vi "RESPALDO.vi"() -> ()   [LabVIEW 2017]
uses:
  <vilib>/myRIO/Instrument Drivers/Onboard IO/PWM/typedefs/PWM Reference.ctl
  <vilib>/myRIO/Common/Instrument Driver Framework/Utilities/typedefs/myRIO Generic Hardware Reference.ctl
  <vilib>/myRIO/Common/Instrument Driver Framework/Utilities/typedefs/Hardware Version Enum.ctl
  <vilib>/myRIO/Common/Instrument Driver Framework/Utilities/typedefs/myRIO v1.0 Reference.ctl
  <vilib>/myRIO/Common/Instrument Driver Framework/Utilities/typedefs/Generic FPGA Reference.ctl
  <vilib>/myRIO/Common/Instrument Driver Framework/myRIO v1.0/PWM/typedefs/PWM Channels Enum.ctl
  <vilib>/myRIO/Instrument Drivers/Onboard IO/PWM/typedefs/PWM Configuration.ctl
  <vilib>/userdefined/High Color/nirio_resource_hc.ctl
  <vilib>/myRIO/Instrument Drivers/Onboard IO/DIO/typedefs/DIO Reference.ctl
  <vilib>/myRIO/Common/Instrument Driver Framework/myRIO v1.0/DIO/typedefs/DIO Channels List.ctl
  <vilib>/myRIO/Common/Instrument Driver Framework/myRIO v1.0/DIO/typedefs/DIO Channels Enum.ctl
  <vilib>/myRIO/Common/Instrument Driver Framework/Utilities/vis/Is FPGA Ref Available.vi
  <vilib>/myRIO/Common/Instrument Driver Framework/myRIO v1.0/DIO/vis/myRIO v1.1 Open DIO.vi
  <vilib>/myRIO/Instrument Drivers/Onboard IO/DIO/vis/Write.vi
  <vilib>/myRIO/Common/Instrument Driver Framework/myRIO v1.0/PWM/vis/myRIO v1.1 Open PWM.vi
  <vilib>/myRIO/Common/Instrument Driver Framework/myRIO v1.0/UART/vis/myRIO v1.0 Close UART.vi
  <vilib>/myRIO/Common/Instrument Driver Framework/Utilities/vis/Validate Channels.vi
  <vilib>/myRIO/Common/Instrument Driver Framework/myRIO v1.0/DIO/vis/myRIO v1.0 Reserve DIO.vi
  <vilib>/myRIO/Common/Instrument Driver Framework/myRIO v1.0/PWM/vis/myRIO v1.0 Reserve PWM.vi
  <vilib>/myRIO/Common/Instrument Driver Framework/myRIO v1.0/Resource Manager/vis/myRIO v1.0 Reserve Channel List.vi
  <vilib>/myRIO/Common/Instrument Driver Framework/myRIO v1.0/DIO/vis/myRIO v1.0 Build MUX Configuration DIO.vi
  <vilib>/myRIO/Common/Instrument Driver Framework/myRIO v1.0/PWM/vis/myRIO v1.0 Build MUX Configuration PWM.vi
  <vilib>/myRIO/Common/Instrument Driver Framework/myRIO v1.0/Resource Manager/vis/myRIO v1.0 Reserve Channel.vi
  <vilib>/myRIO/Common/Instrument Driver Framework/myRIO v1.0/Resource Manager/vis/myRIO v1.0 Unreserve Channel.vi
  <vilib>/myRIO/Common/Instrument Driver Framework/myRIO v1.0/Resource Manager/vis/myRIO v1.0 Create Configuration List.vi
  <vilib>/myRIO/Common/Instrument Driver Framework/myRIO v1.0/Resource Manager/vis/myRIO v1.0 Build Mutex Name.vi
  <vilib>/Utility/VariantDataType/GetNumericInfo.vi
  <vilib>/Utility/error.llb/Error Cluster From Error Code.vi
  <vilib>/myRIO/Common/Instrument Driver Framework/myRIO v1.0/myRIO v1.1 Open.vi
  <vilib>/myRIO/Common/Instrument Driver Framework/Utilities/vis/IO Manager.vi
  <vilib>/myRIO/Common/Instrument Driver Framework/Utilities/vis/Configuration Manager.vi
  <vilib>/myRIO/Common/Instrument Driver Framework/myRIO v1.0/Resource Manager/vis/myRIO v1.0 Configure IO.vi
  <vilib>/myRIO/Common/Instrument Driver Framework/myRIO v1.0/myRIO v1.0 Close.vi
  <vilib>/myRIO/Common/Instrument Driver Framework/myRIO v1.0/PWM/vis/myRIO v1.0 Write PWM.vi
  <vilib>/myRIO/Common/Instrument Driver Framework/myRIO v1.0/DIO/vis/myRIO v1.0 Write DIO.vi
  <vilib>/myRIO/Common/Instrument Driver Framework/Utilities/vis/FPGA Ref Manager.vi
  <vilib>/myRIO/Common/Instrument Driver Framework/myRIO v1.0/myRIO v1.0 Reset FPGA.vi
  <vilib>/myRIO/Common/Instrument Driver Framework/myRIO v1.0/IRQ/vis/myRIO v1.0 IRQ Info FGV.vi
  <vilib>/myRIO/Common/Instrument Driver Framework/myRIO v1.0/IRQ/vis/myRIO v1.0 Timer IRQ Info FGV.vi
  <vilib>/myRIO/Common/Instrument Driver Framework/myRIO v1.0/IRQ/vis/myRIO v1.0 ISR Agent.vi
  <vilib>/myRIO/Express VI/Onboard IO/PWM/PWM Express VI.xnode
  <vilib>/myRIO/Instrument Drivers/Onboard IO/PWM/vis/myRIO PWM Open.xnode
  <vilib>/myRIO/Express VI/Onboard IO/DO/DO Express VI.xnode
  <vilib>/myRIO/Instrument Drivers/Onboard IO/DIO/vis/myRIO DIO Open.xnode
  <vilib>/myRIO/Instrument Drivers/Utilities/Utilities.lvlib
  <vilib>/myRIO/Instrument Drivers/Onboard IO/PWM/PWM.lvlib
  <vilib>/myRIO/Instrument Drivers/Onboard IO/DIO/DIO.lvlib
panel:
  in  "delta":dbl
  in  "Numeric 7":dbl
  in  "Numeric 6":dbl
  out "Numeric 5":dbl
  out "Numeric 4":dbl
  out "Numeric 3":dbl
  in  "MODO JOG":bool
  out "Numeric 2":dbl
  out "Slide 2":dbl(slide) scale=-200.0..100.0
  out "Slide":dbl(slide) scale=-200.0..100.0
  out "Numeric":dbl
  in  "control":T1(tab)
  in  "PARADA":bool
  out "ESTADO":string
  in  "?":bool
  out "MODO":string
  in  "Boolean":bool
  in  "PWM channel":tag="B/PWM0"
  in  "PWM channel 2":tag="B/PWM0"
  out "offset [%FS] 3":dbl
  in  "null offset 3":bool
  out "duty cycle [%] 3":dbl
  out "pulse width [ms] 3":dbl=1.5
  in  "position 2":dbl(slide) scale=-200.0..200.0
  in  "PWM channel 3":tag="B/PWM0"
  out "offset [%FS] 4":dbl
  in  "null offset 4":bool
  out "duty cycle [%] 4":dbl
  out "pulse width [ms] 4":dbl=1.5
  in  "position [%FS] 4":dbl(slide) scale=-200.0..200.0
  out "offset [%FS] 5":dbl
  in  "null offset 5":bool
  out "duty cycle [%] 5":dbl
  out "pulse width [ms] 5":dbl=1.5
  in  "position [%FS] 5":dbl(slide) scale=-200.0..200.0
  out "position [%FS]":dbl
  out "position [3":dbl
  out "position1":dbl
  out "ventosa":bool
  out "POSICION1":dbl
  out "POSICION2":dbl
  out "POSICION3":dbl
  in  "velocidad":dbl(knob) scale=20.0..250.0
  in  "PARADA":bool
  out "INDICADOR 2":bool
  out "INDICADOR1":bool
  in  "PARADA":bool
  in  ".":dbl(slide) scale=0.0..10.0
  in  ".":dbl(slide) scale=0.0..10.0
  out "String":string
  out "CADENA1":dbl
  out "CADENA2":dbl
  in  "Puero de servicio remoto":u16
  in  "direccion":string
  in  "PARADA":bool
  out "Datos recibidos vía TCP":cluster{dbl, dbl}(graph)
  out "offset [%FS] 2":dbl
  in  "null offset 2":bool
  out "duty cycle [%] 2":dbl
  out "pulse width [ms] 2":dbl=1.5
  in  "freq [Hz] 2":dbl=50.0
  in  "position [%FS] 3":dbl(slide) scale=-400.0..400.0
  in  "PWM channel 6":tag="B/PWM0"
  in  "PWM channel 5":tag="B/PWM0"
  in  "position [%FS] 2":dbl(slide) scale=-400.0..400.0
  in  "freq [Hz]":dbl=50.0
  out "pulse width [ms]":dbl=1.5
  out "duty cycle [%]":dbl
  in  "null offset":bool
  out "offset [%FS]":dbl
  out "offset [%FS] 6":dbl
  in  "null offset 6":bool
  out "duty cycle [%] 6":dbl
  out "pulse width [ms] 6":dbl=1.5
  in  "freq [Hz] 3":dbl=50.0
  in  "position [%FS] 6":dbl(slide) scale=-400.0..400.0
  in  "PWM channel 7":tag="B/PWM0"
  in  "VELOCIDAD1":dbl(knob) scale=0.0..1.0
  in  "VELOCIDAD 2":dbl(knob) scale=0.0..1.0
  in  "DIRECCION1":bool
  in  "DIRECCION 2":bool
  in  "servomotores":bool
  out "V1":dbl
  out "V2":dbl
  # "BIENVENIDOS A LA\nINTERFAZ DE CONTROL ROBOT DELTA"
  # "INICIO DE PROCESO"
  # "SISTEMA DE ESTADO DE ROBOT DELTA"
  # "SERVOMOTOR1"
  # "SERVOMOTOR2"
  # "SERVOMOTOR3"
  # "VISUALIZACION DE CINTAS TRANSPORTADORAS"
  # "CINTA TRANSPORTADORA1"
  # "CINTA TRANSPORTADORA2"
  # "COMUNICACION CON EL SISTEMA DE VISION"
  # "DATOS DE COMIUNICACION"
  # "VISUALIZACION DE POSCICION"
  # "SERVOMOTOR1"
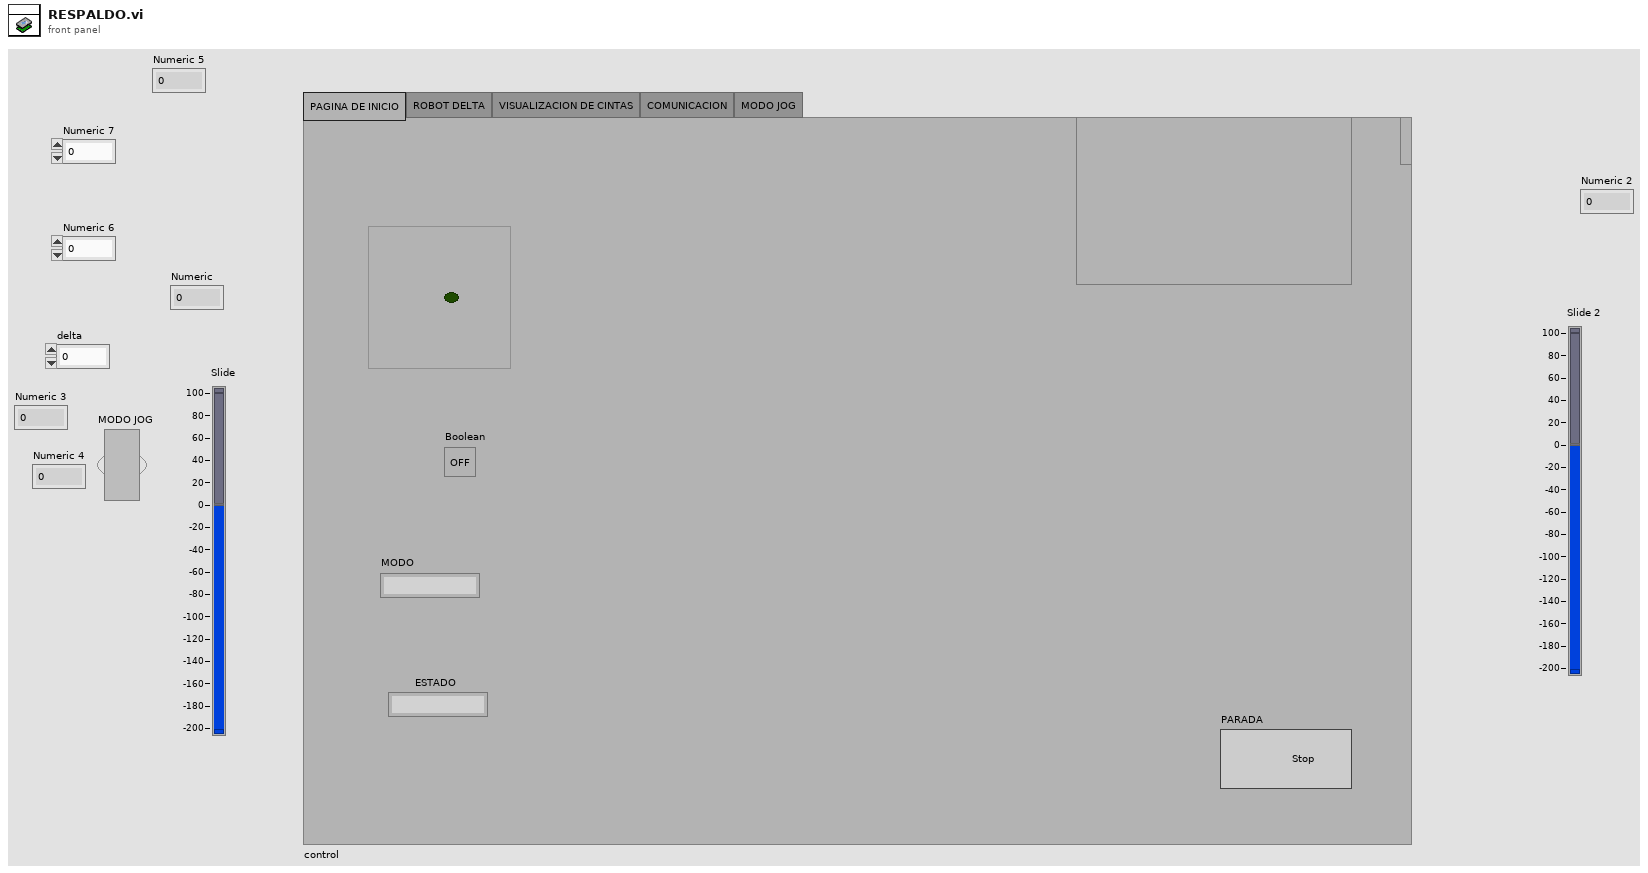
[diagram p1: front panel]
types:
  T1 = enum32{"PAGINA DE INICIO", "ROBOT DELTA", "VISUALIZACION DE CINTAS", "COMUNICACION", "MODO JOG"}
  T2 = enum16{"", "INICIO", "STOP", "DETECCION", "ESPERA", "MOVIMIENTO"}
  T3 = typedef "PWM.lvlib/PWM Reference.ctl" = cluster{"myRIO Reference":T4, "PWM Channels Enum":T8, "PWM Configuration":T9}
  T4 = typedef "myRIO Generic Hardware Reference.ctl" = cluster{"myRIO Model":T5, "myRIO Hardware Reference":T6}
  T5 = typedef "Hardware Version Enum.ctl" = enum16{"Unknown", "myRIO-1900", "myRIO-1950", "roboRIO", "NI ELVIS RIO CM"}
  T6 = typedef "myRIO v1.0 Reference.ctl" = cluster{"Generic FPGA Reference":T7, "Allow multiple opens":bool}
  T7 = typedef "Generic FPGA Reference.ctl" = refnum<k20>
  T8 = typedef "PWM Channels Enum.ctl" = enum16{"Not Connected", "C/PWM0", "C/PWM1", "A/PWM0", "A/PWM1", "A/PWM2", "B/PWM0", "B/PWM1", "B/PWM2", "PWM/PWM0", "PWM/PWM1", "PWM/PWM2", "PWM/PWM3", "PWM/PWM4", "PWM/PWM5", "PWM/PWM6", "PWM/PWM7", "PWM/PWM8", "PWM/PWM9"}
  T9 = typedef "PWM.lvlib/PWM Configuration.ctl" = cluster{"Frequency":dbl, "Duty Cycle":dbl}
  T10 = enum16{"Standard", "Buffered", "CRLF", "Immediate"}
  T11 = typedef "nirio_resource_hc.ctl" = tag
  T12 = typedef "DIO.lvlib/DIO Reference.ctl" = cluster{"myRIO Reference":T4, "DIO Channels List":T13}
  T13 = typedef "DIO Channels List.ctl" = T14[]
  T14 = typedef "DIO Channels Enum.ctl" = enum16{"Not Connected", "C/DIO0", "C/DIO1", "C/DIO2", "C/DIO3", "C/DIO4", "C/DIO5", "C/DIO6", "C/DIO7", "A/DIO0", "A/DIO1", "A/DIO2", "A/DIO3", "A/DIO4", "A/DIO5", "A/DIO6", "A/DIO7", "A/DIO8", "A/DIO9", "A/DIO10", "A/DIO11", "A/DIO12", "A/DIO13", "A/DIO14", "A/DIO15", "B/DIO0", "B/DIO1", "B/DIO2", "B/DIO3", "B/DIO4", "B/DIO5", "B/DIO6", "B/DIO7", "B/DIO8", "B/DIO9", "B/DIO10", "B/DIO11", "B/DIO12", "B/DIO13", "B/DIO14", "B/DIO15", "LED0", "LED1", "LED2", "LED3", "Button0", "DIO/DIO0", "DIO/DIO1", "DIO/DIO2", "DIO/DIO3", "DIO/DIO4", "DIO/DIO5", "DIO/DIO6", "DIO/DIO7", "DIO/DIO8", "DIO/DIO9", "SPI/CS0", "SPI/CS1", "SPI/CS2", "SPI/CS3", "LED RADIO (Green)", "LED RADIO (Red)", "LED COMM (Green)", "LED COMM (Red)", "LED MODE (Green)", "LED MODE (Red)"}
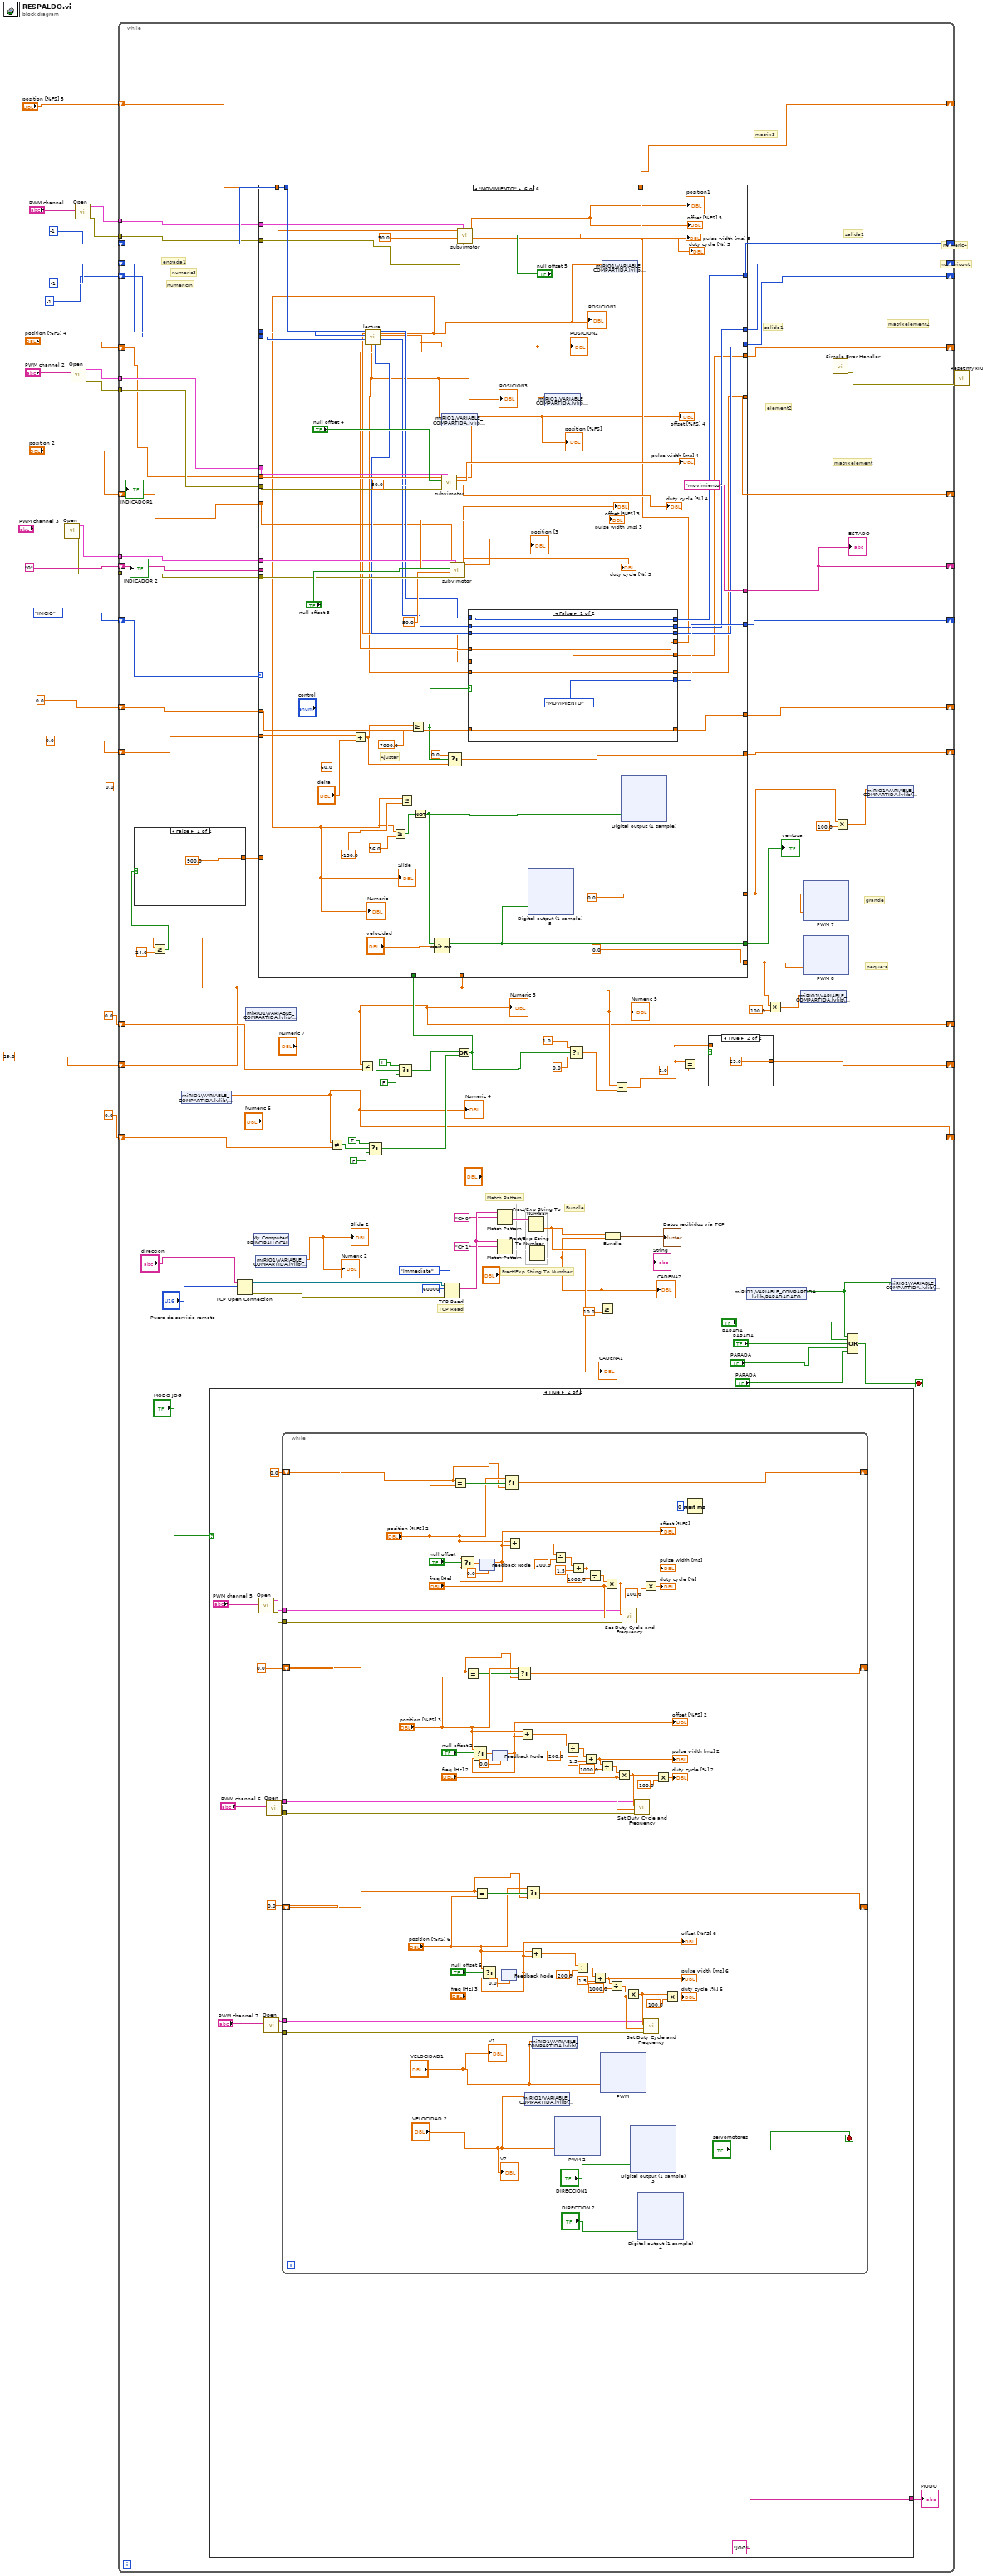
[diagram p0: block diagram]
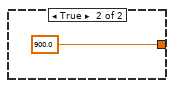
[diagram p2: hidden frame]
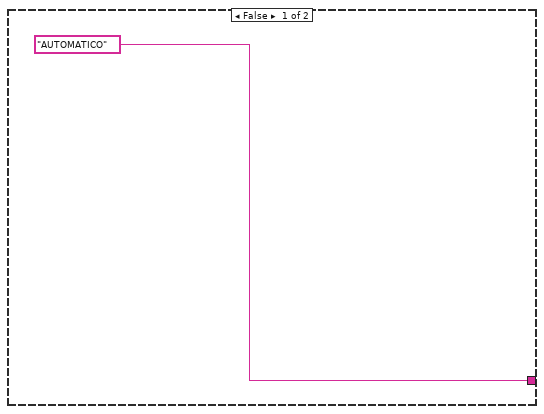
[diagram p4: hidden frame]
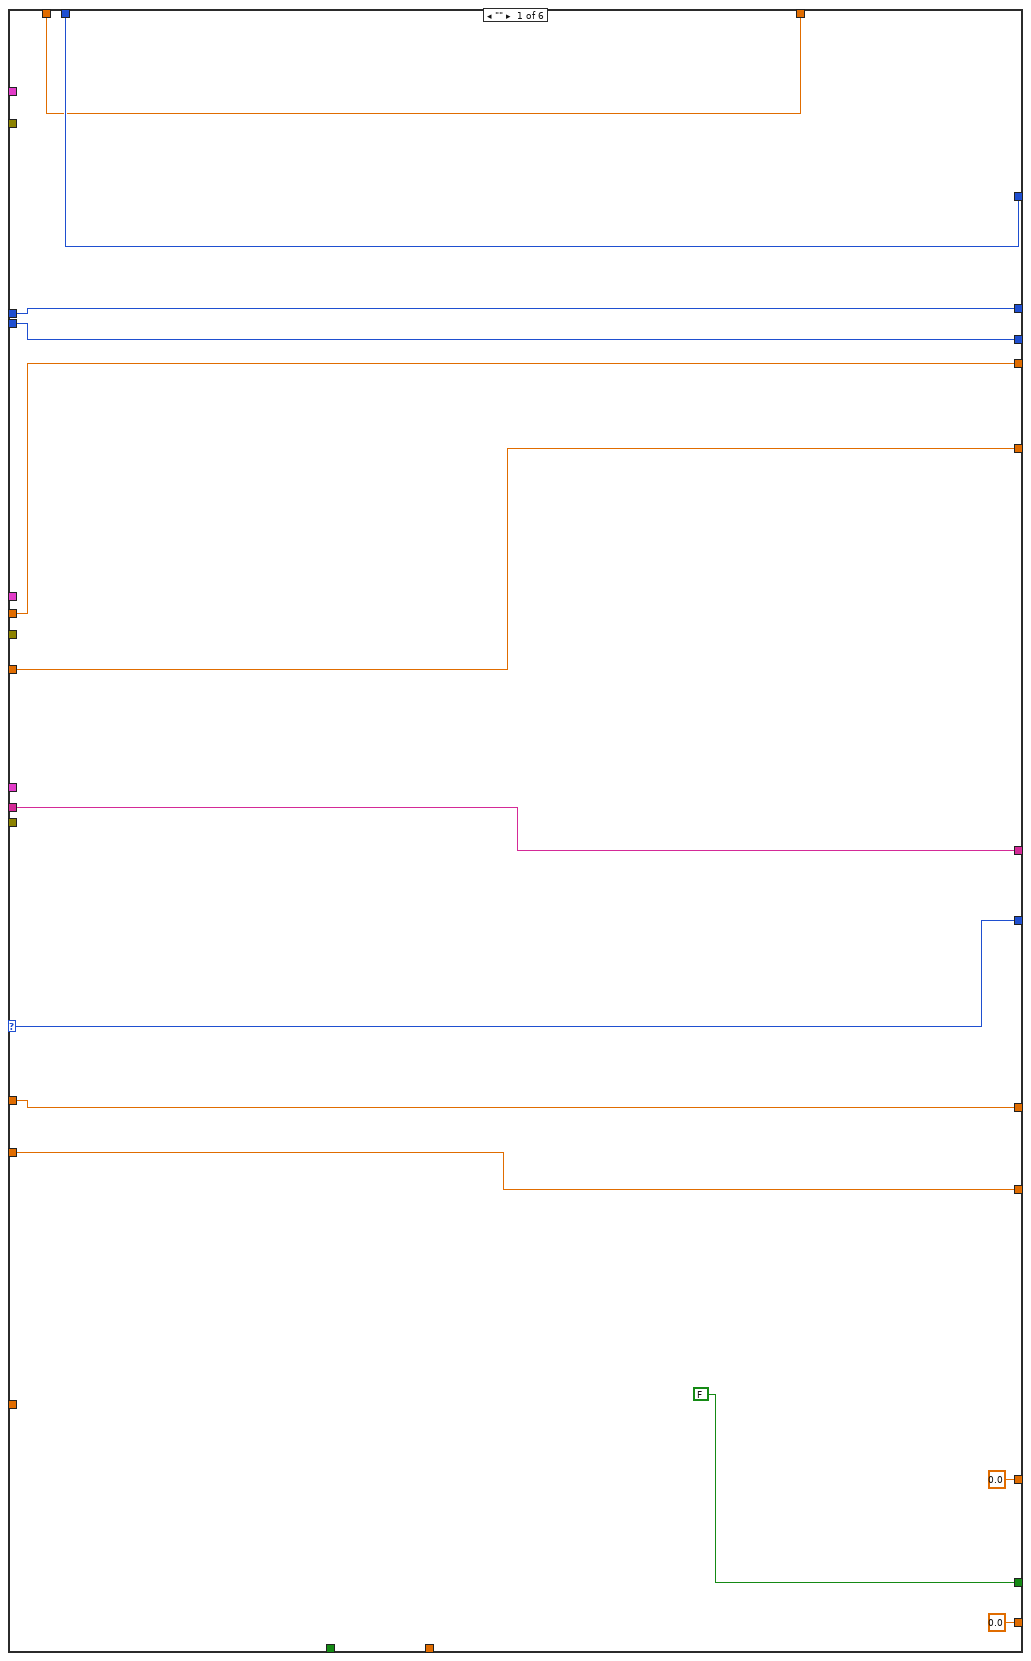
[diagram p5: hidden frame]
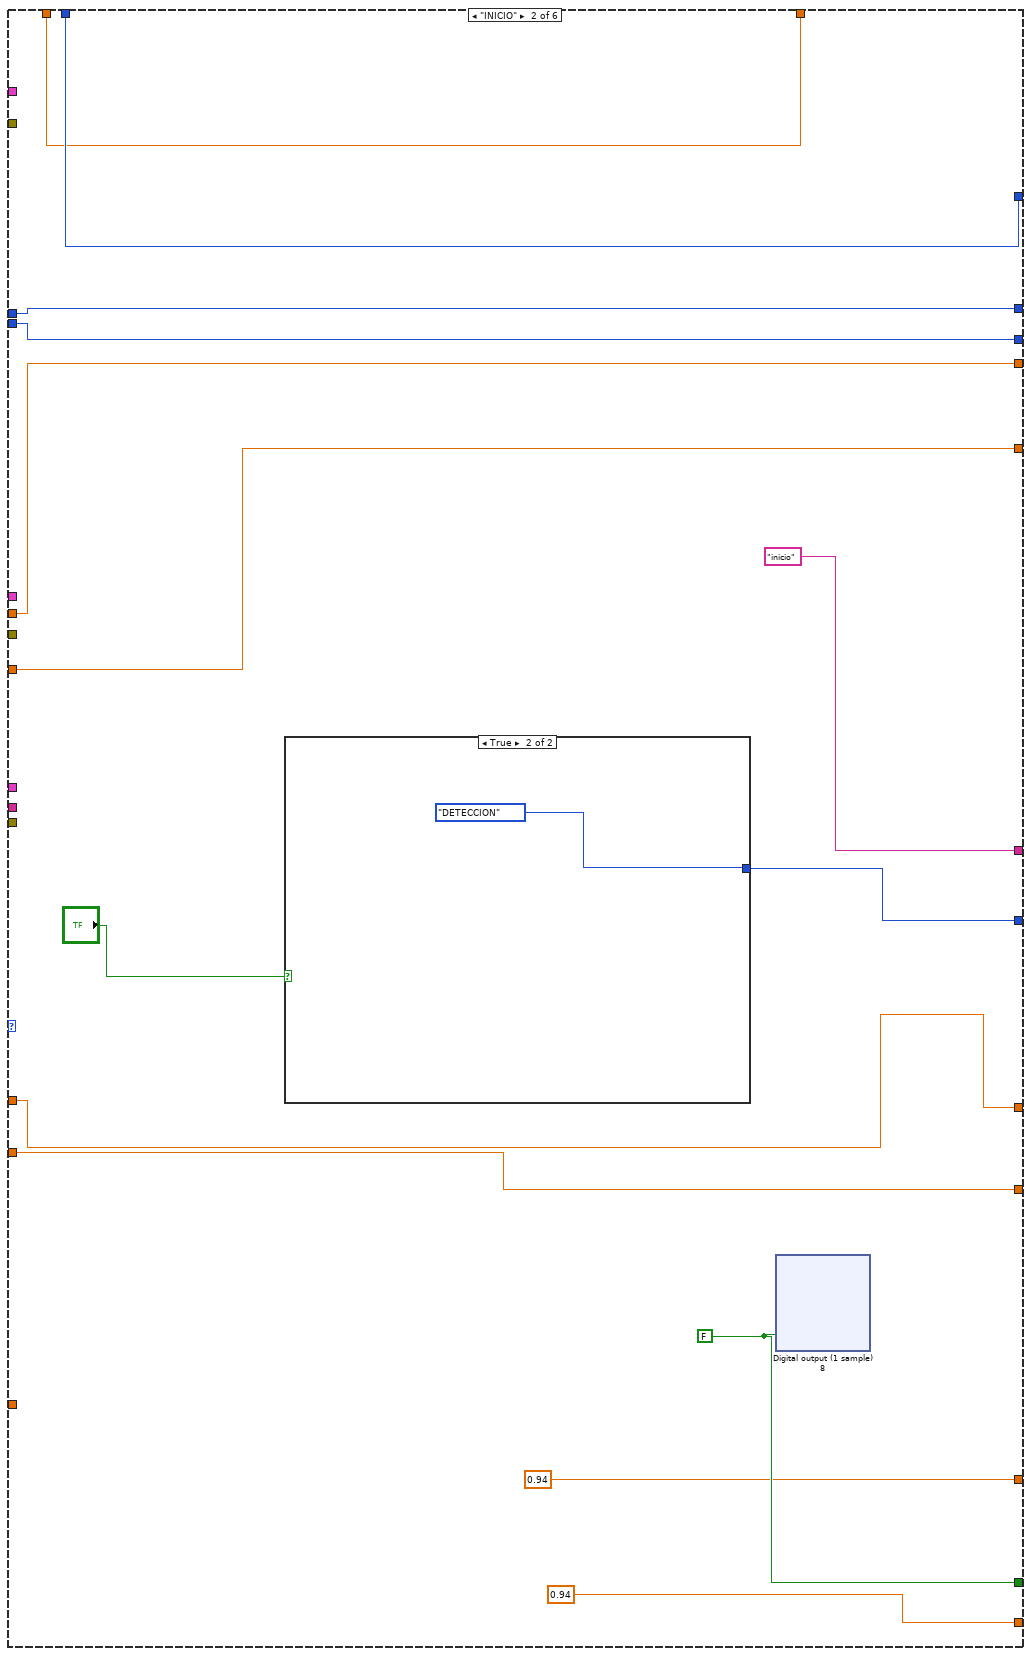
[diagram p6: hidden frame]
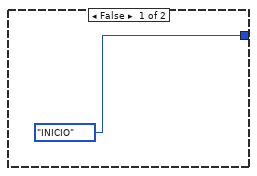
[diagram p7: hidden frame]
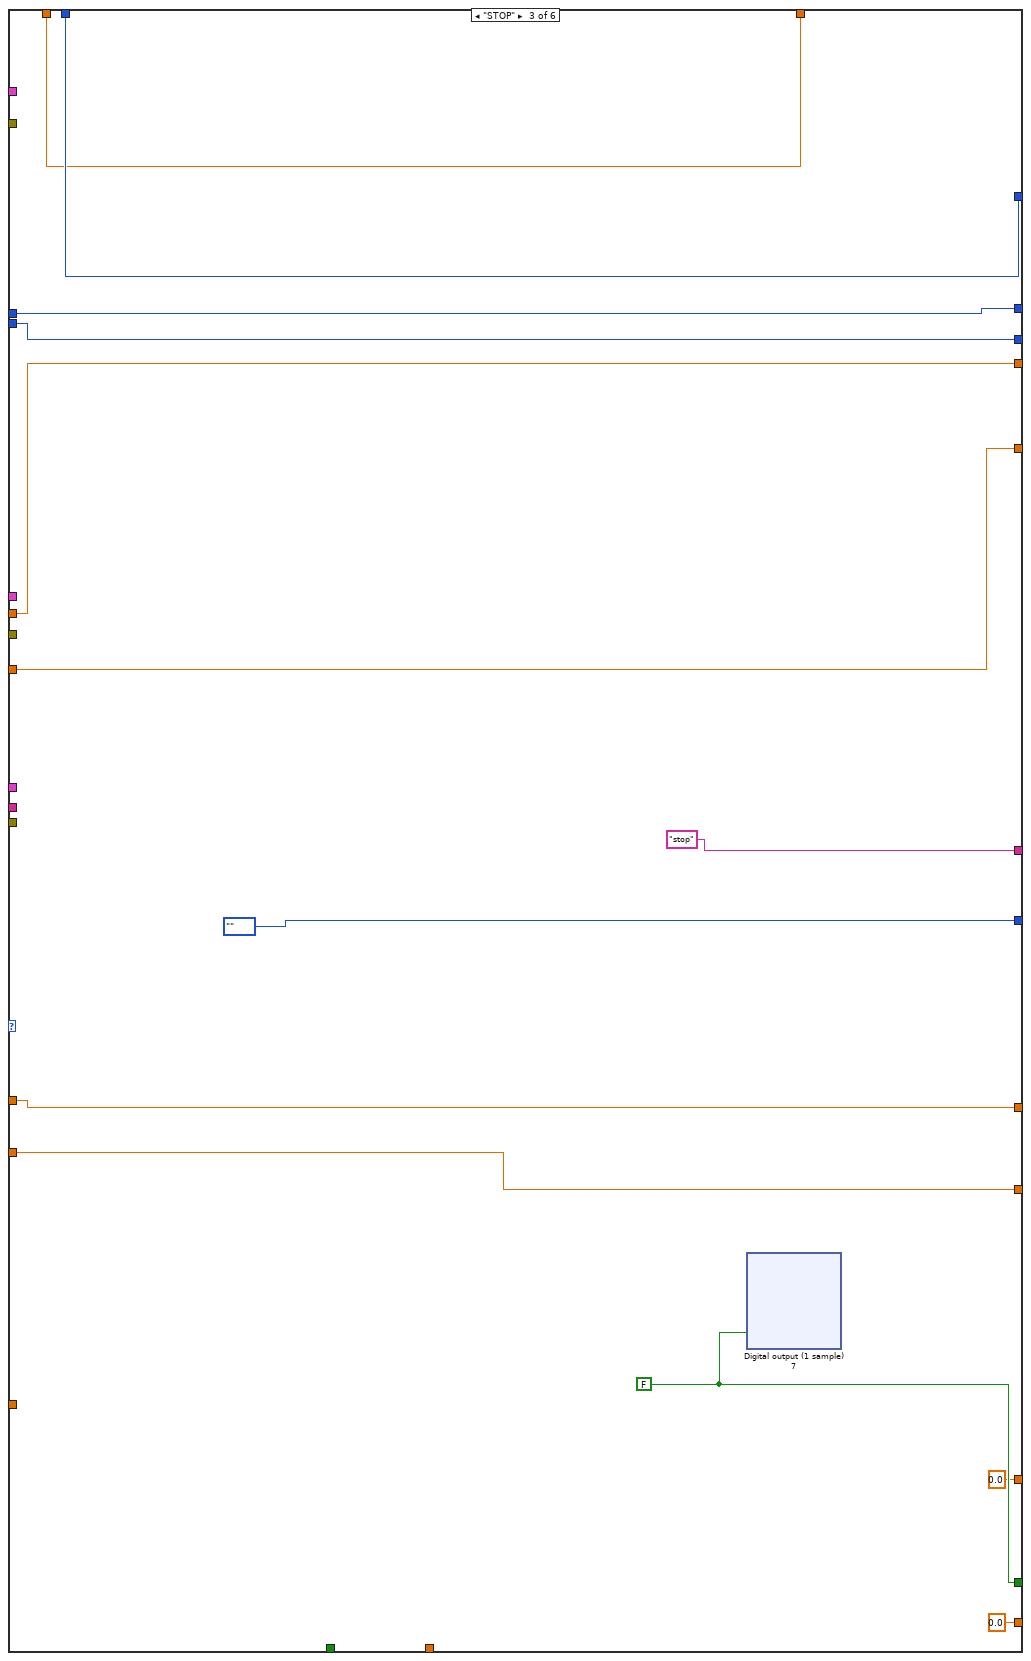
[diagram p8: hidden frame]
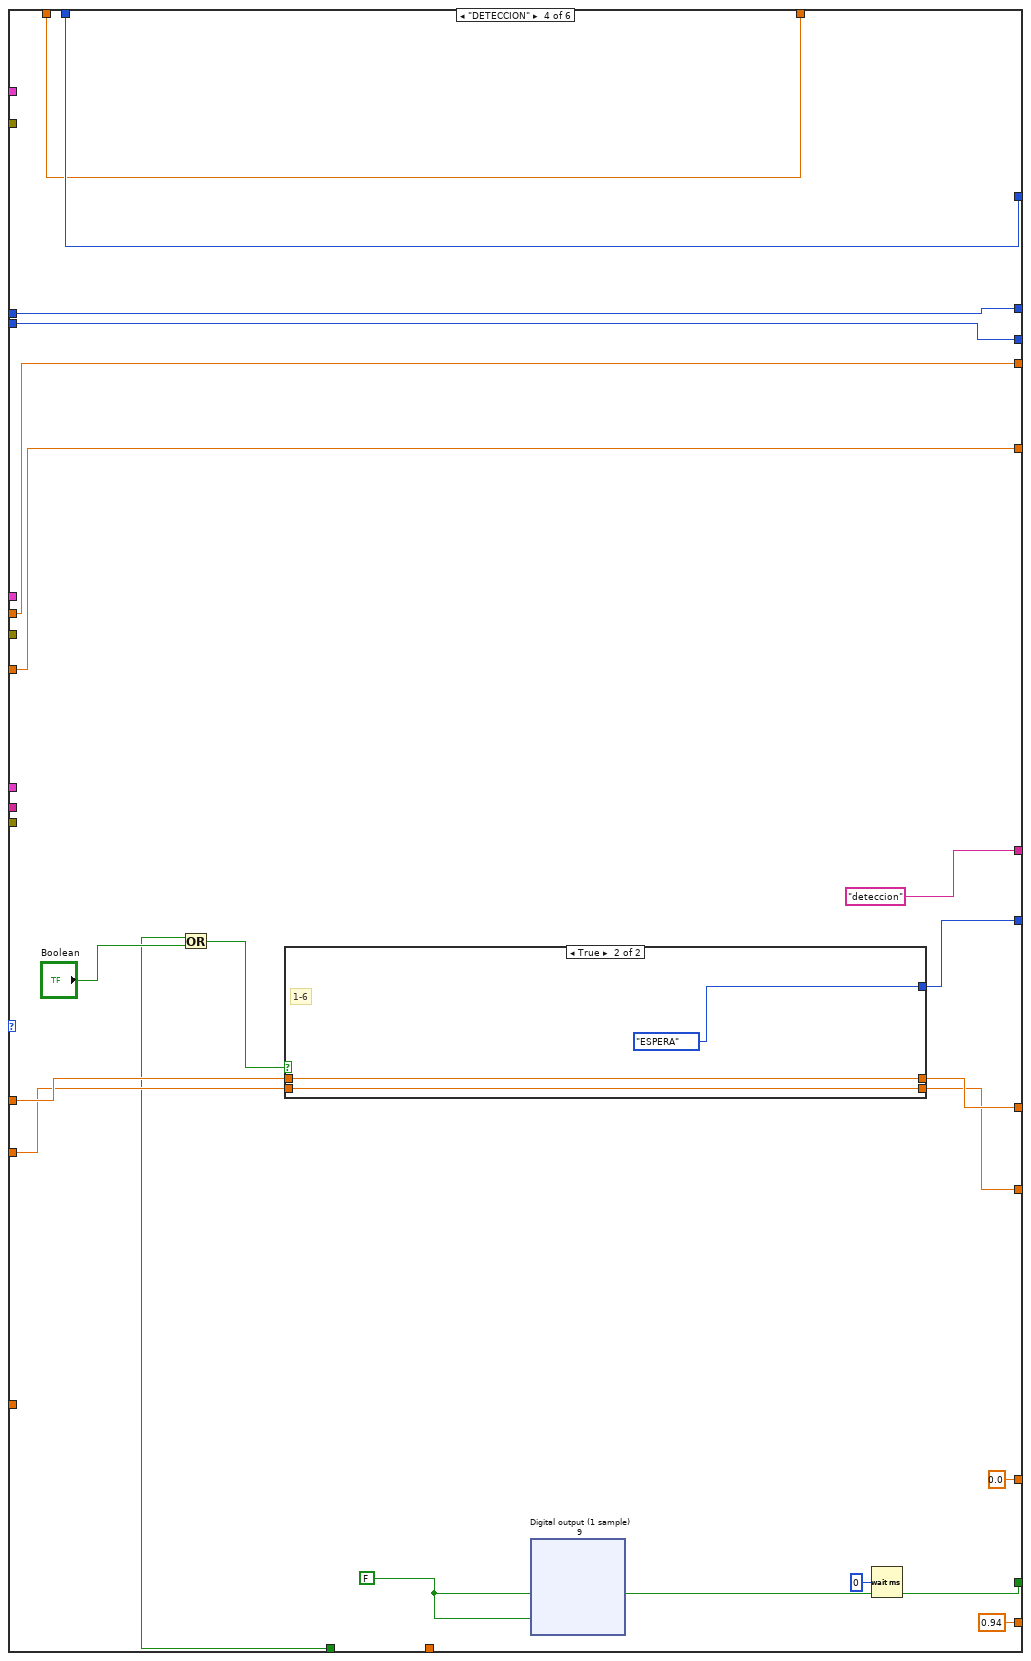
[diagram p9: hidden frame]
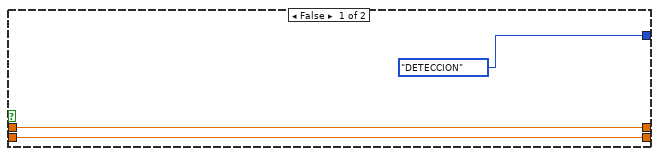
[diagram p10: hidden frame]
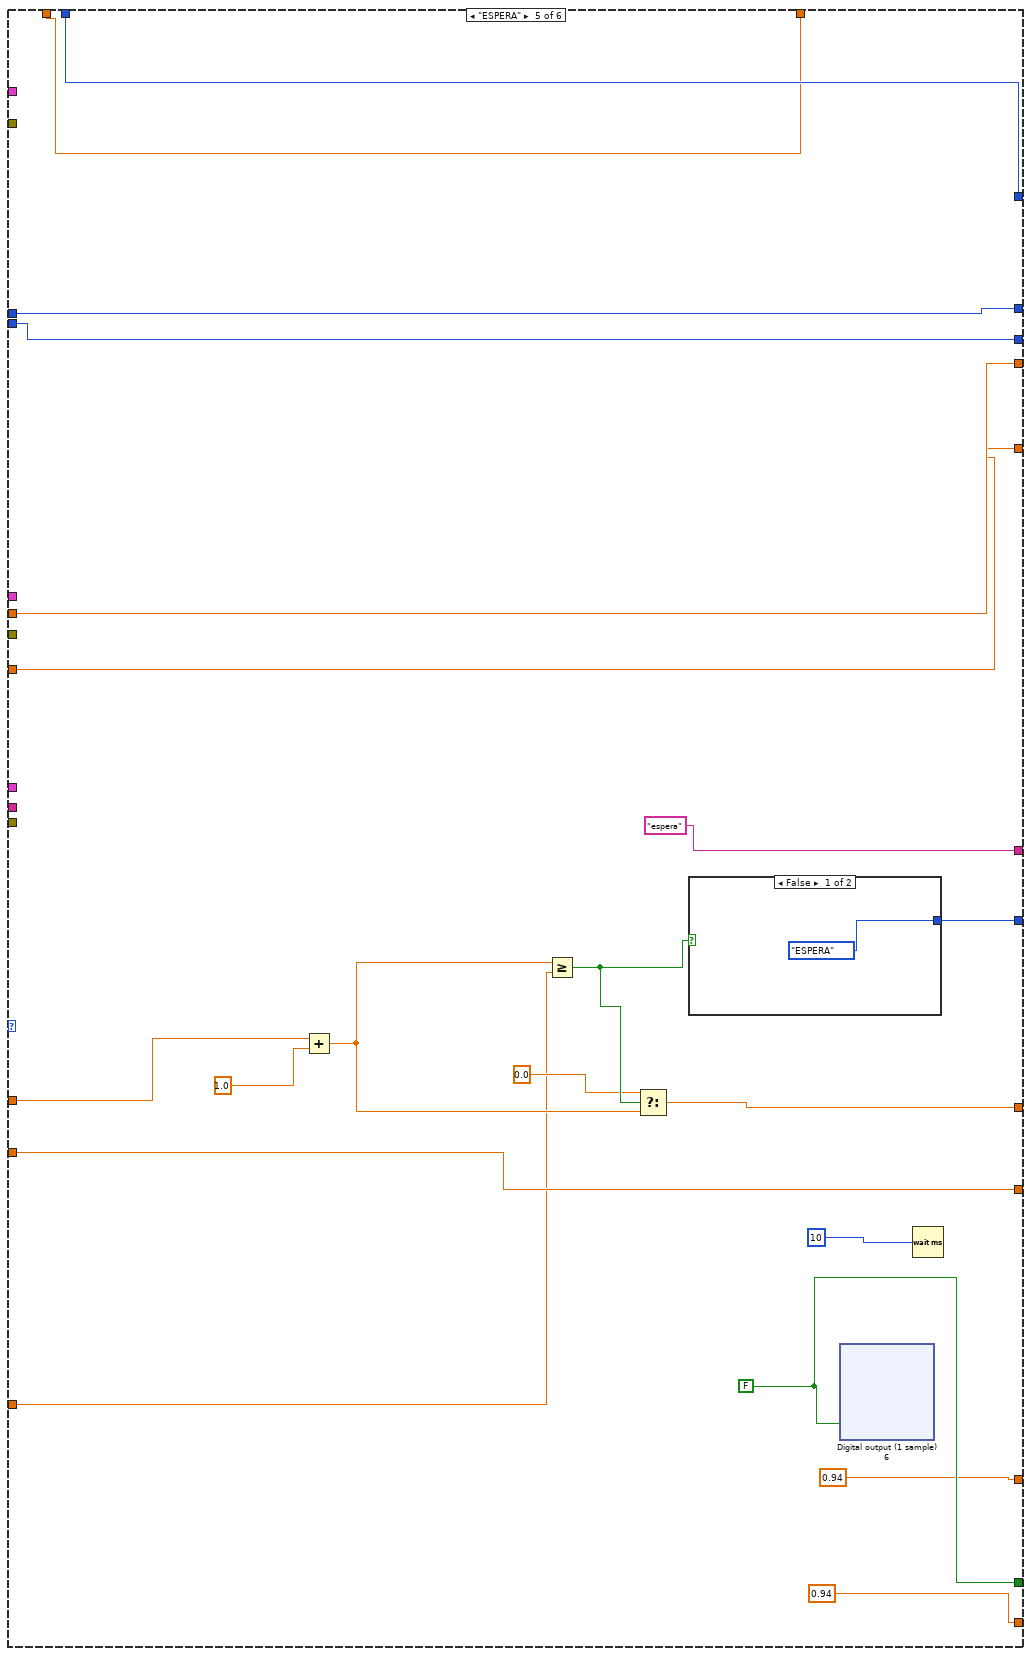
[diagram p11: hidden frame]
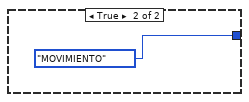
[diagram p12: hidden frame]
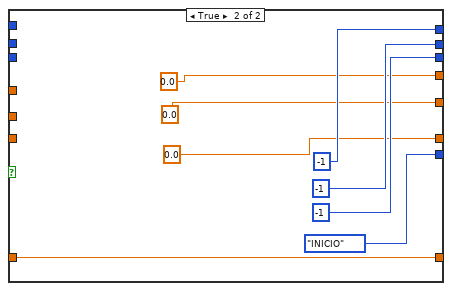
[diagram p13: hidden frame]
diagram:
  (unwired) 0.0
  # "numericout"
  # "numeric4"
  # "salida1"
  n1 = call <vilib>:"Open.vi"("Channel Name"="PWM channel 3") -> ("error out"=w11:errorcluster, "PWM Ref Out"=w12:T3)  [unwired: 9 in]
  n2 = call <vilib>:"Open.vi"("Channel Name"="PWM channel 2") -> ("error out"=w8:errorcluster, "PWM Ref Out"=w9:T3)  [unwired: 9 in]
  n3 = call <vilib>:"Open.vi"("Channel Name"="PWM channel") -> ("error out"=w5:errorcluster, "PWM Ref Out"=w6:T3)  [unwired: 9 in]
  n4 = while {
    shift-right: [w87] -> _
    shift-left: -1 -> [w91]
    shift-right: [w85] -> _
    shift-left: -1 -> [w90]
    shift-right: [w84] -> _
    shift-left: -1 -> [w89]
    shift-right: [w88] -> _
    shift-left: "position [%FS] 5" -> [w80]
    shift-right: [w86] -> _
    shift-left: "position [%FS] 4" -> [w92]
    shift-right: [w83] -> _
    shift-left: "position 2" -> [w95]
    shift-right: [w103] -> _
    shift-left: T2."INICIO" -> [w104]
    shift-right: [w102] -> _
    shift-left: 0.0 -> [w101]
    shift-right: [w100] -> _
    shift-left: 0.0 -> [w79]
    shift-right: [w99] -> _
    shift-left: "0" ("String") -> [w98]
    tunnel: w12 -> [w97]
    tunnel: w11 -> [w96]
    tunnel: w9 -> [w94]
    tunnel: w8 -> [w93]
    tunnel: w6 -> [w82]
    tunnel: w5 -> [w81]
    shift-right: [w50] -> _
    shift-left: 29.0 ("f") -> [w35]
    shift-right: [w31] -> _
    shift-left: 0.0 ("Double") -> [w46]
    shift-right: [w32] -> _
    shift-left: 0.0 ("Double") -> [w38]
    stop <- w56 stop-if-true
    # "grande"
    # "peque;a"
    # "matrixelement2"
    # "matrixelement"
    # "Bundle"
    # "TCP Read"
    # "Fract/Exp String To Number"
    # "Match Pattern"
    # "element2"
    # "salida1"
    # "matrix3"
    # "numericin"
    # "numeric3"
    # "entrada1"
    n5 = Greater Or Equal?(x=w35, y=24.0) -> (x >= y?=w36:bool)
    n6 = case shown="False" w36 {
      tunnel: [900.0 ("y") 900.0 ("y")] -> w33
      frame False {
      }
      frame True {
      }
    }
    n7 = shared-variable "miRIO1\\VARIABLE_COMPARTIDA.lvlib\\POSICION2"() -> (w31:dbl)  [unwired: 1 in, 1 out]
    "Numeric 4" <- w31
    n8 = case shown="True" "MODO JOG" {
      tunnel: ["AUTOMATICO" ("MODO") "JOG" ("MODO")] -> w30
      frame False {
      }
      frame True {
        n9 = call <vilib>:"Open.vi"("Channel Name"="PWM channel 5") -> ("error out"=w190:errorcluster, "PWM Ref Out"=w191:T3)  [unwired: 9 in]
        n10 = call <vilib>:"Open.vi"("Channel Name"="PWM channel 7") -> ("error out"=w184:errorcluster, "PWM Ref Out"=w185:T3)  [unwired: 9 in]
        n11 = call <vilib>:"Open.vi"("Channel Name"="PWM channel 6") -> ("error out"=w187:errorcluster, "PWM Ref Out"=w188:T3)  [unwired: 9 in]
        n12 = while {
          tunnel: w191 -> [w243]
          tunnel: w190 -> [w242]
          shift-right: [w241] -> _
          shift-left: 0.0 ("position [%FS] 2") -> [w240]
          shift-right: [w221] -> _
          shift-left: 0.0 ("position [%FS] 3") -> [w222]
          tunnel: w188 -> [w220]
          tunnel: w187 -> [w219]
          shift-right: [w200] -> _
          shift-left: 0.0 ("position [%FS] 6") -> [w201]
          tunnel: w185 -> [w199]
          tunnel: w184 -> [w198]
          stop <- "servomotores" stop-if-true
          n13 = Equal?(x=w240, y="position [%FS] 2") -> (x = y?=w245:bool)
          n14 = Equal?(x=w222, y="position [%FS] 3") -> (x = y?=w238:bool)
          n15 = Equal?(x=w201, y="position [%FS] 6") -> (x = y?=w203:bool)
          n16 = feedback #1(0.0 ("position [%FS]")) -> (w251:dbl)
          "offset [%FS]" <- w251
          n17 = Select(t="position [%FS] 2", s="null offset", f=w251) -> (s? t:f=w253:dbl)
          n18 = feedback-in #1(w253) -> ()
          n19 = feedback #2(0.0 ("position [%FS]")) -> (w232:dbl)
          "offset [%FS] 2" <- w232
          n20 = Select(t="position [%FS] 3", s="null offset 2", f=w232) -> (s? t:f=w230:dbl)
          n21 = feedback-in #2(w230) -> ()
          n22 = feedback #3(0.0 ("position [%FS]")) -> (w209:dbl)
          "offset [%FS] 6" <- w209
          n23 = Select(t="position [%FS] 6", s="null offset 6", f=w209) -> (s? t:f=w211:dbl)
          n24 = feedback-in #3(w211) -> ()
          n25 = Select(t="position [%FS] 2", s=w245, f=w240) -> (s? t:f=w241:dbl)
          n26 = Add(x="position [%FS] 2", y=w251) -> (x+y=w252:dbl)
          n27 = Select(t="position [%FS] 3", s=w238, f=w222) -> (s? t:f=w221:dbl)
          n28 = Add(x="position [%FS] 3", y=w232) -> (x+y=w231:dbl)
          n29 = shared-variable "miRIO1\\VARIABLE_COMPARTIDA.lvlib\\MOTOR2"("VELOCIDAD 2") -> ()  [unwired: 1 in, 1 out]
          n30 = Select(t="position [%FS] 6", s=w203, f=w201) -> (s? t:f=w200:dbl)
          n31 = Add(x="position [%FS] 6", y=w209) -> (x+y=w210:dbl)
          n32 = shared-variable "miRIO1\\VARIABLE_COMPARTIDA.lvlib\\MOTOR1"("VELOCIDAD1") -> ()  [unwired: 1 in, 1 out]
          n33 = Divide(x=w252, y=200.0) -> (x/y=w259:dbl)
          n34 = xnode "PWM 2"("Duty Cycle"="VELOCIDAD 2") -> ()  [unwired: 1 in, 1 out]
          n35 = Divide(x=w231, y=200.0) -> (x/y=w224:dbl)
          n36 = Add(x=w259, y=1.5) -> (x+y=w257:dbl)
          "pulse width [ms]" <- w257
          n37 = Divide(x=w210, y=200.0) -> (x/y=w217:dbl)
          n38 = Add(x=w224, y=1.5) -> (x+y=w226:dbl)
          "pulse width [ms] 2" <- w226
          n39 = Divide(x=w257, y=1000.0) -> (x/y=w250:dbl)
          n40 = Add(x=w217, y=1.5) -> (x+y=w215:dbl)
          "pulse width [ms] 6" <- w215
          n41 = Divide(x=w226, y=1000.0) -> (x/y=w233:dbl)
          n42 = xnode "PWM"("Duty Cycle"="VELOCIDAD1") -> ()  [unwired: 1 in, 1 out]
          n43 = Multiply(x=w250, y="freq [Hz]") -> (x*y=w247:dbl)
          n44 = Divide(x=w215, y=1000.0) -> (x/y=w208:dbl)
          n45 = Multiply(x=w233, y="freq [Hz] 2") -> (x*y=w236:dbl)
          n46 = call <vilib>:"Set Duty Cycle and Frequency.vi"("error in (no error)"=w242, "Frequency [Hz]"="freq [Hz]", "Duty Cycle"=w247, "PWM Ref In"=w243) -> ()  [unwired: 5 in, 2 out]
          n47 = Multiply(x=w208, y="freq [Hz] 3") -> (x*y=w205:dbl)
          n48 = xnode "Digital output (1 sample) 3"("B/DIO0 (Pin 11)"="DIRECCION1") -> ()  [unwired: 1 in, 1 out]
          n49 = call <vilib>:"Set Duty Cycle and Frequency.vi"("error in (no error)"=w219, "Frequency [Hz]"="freq [Hz] 2", "Duty Cycle"=w236, "PWM Ref In"=w220) -> ()  [unwired: 5 in, 2 out]
          n50 = xnode "Digital output (1 sample) 4"("B/DIO1 (Pin 13)"="DIRECCION 2") -> ()  [unwired: 1 in, 1 out]
          n51 = Multiply(x=w247, y=100.0) -> (x*y=→"duty cycle [%]":dbl)
          n52 = call <vilib>:"Set Duty Cycle and Frequency.vi"("error in (no error)"=w198, "Frequency [Hz]"="freq [Hz] 3", "Duty Cycle"=w205, "PWM Ref In"=w199) -> ()  [unwired: 5 in, 2 out]
          n53 = Multiply(x=w236, y=100.0) -> (x*y=→"duty cycle [%] 2":dbl)
          n54 = Multiply(x=w205, y=100.0) -> (x*y=→"duty cycle [%] 6":dbl)
          n55 = Wait (ms)(milliseconds to wait=u32 0) -> ()  [unwired: 1 out]
          "V1" <- "VELOCIDAD1"
          "V2" <- "VELOCIDAD 2"
        }
      }
    }
    "MODO" <- w30
    n56 = TCP Open Connection(address="direccion", remote port or service name="Puero de servicio remoto") -> (connection ID=w78:refnum<k5>, error out=w77:errorcluster)  [unwired: 3 in]
    n57 = shared-variable "miRIO1\\VARIABLE_COMPARTIDA.lvlib\\POSICION1"() -> (w32:dbl)  [unwired: 1 in, 1 out]
    "Numeric 3" <- w32
    n58 = shared-variable "My Computer\\PRINCIPALLOCAL1.lvlib\\POS1"() -> ()  [unwired: 1 in, 2 out]
    n59 = shared-variable "miRIO1\\VARIABLE_COMPARTIDA.lvlib\\POSICION1"() -> (→"Slide 2" →"Numeric 2":dbl)  [unwired: 1 in, 1 out]
    n60 = Not Equal?(x=w31, y=w46) -> (x != y?=w47:bool)
    n61 = Not Equal?(x=w32, y=w38) -> (x != y?=w39:bool)
    n62 = Select(t=TRUE, s=w47, f=FALSE) -> (s? t:f=w43:bool)
    n63 = Select(t=TRUE, s=w39, f=FALSE) -> (s? t:f=w37:bool)
    n64 = TCP Read(connection ID=w78, bytes to read=60000, error in (no error)=w77, 7:T10."Immediate" ("mode (standard)")) -> (data out=w74:string)  [unwired: 1 in, 2 out]
    n65 = Or(x=w37, y=w43) -> (x .or. y?=w42:bool)
    n66 = case shown="\"MOVIMIENTO\"" w104 {
      selector: w104 -> [w414 _ _ _ _ _]
      tunnel: [w414 w428 T2."" w532 w591 w686] -> w103
      tunnel: [w413 w427 w477 w531 w588 w685] -> w102
      tunnel: w101 -> [w413 w427 w477 w530 w592 w684]
      tunnel: [w412 w426 w476 w529 w590 w679] -> w100
      tunnel: w79 -> [w412 w426 w476 w528 w590 w646]
      tunnel: [w411 "inicio" ("String") "stop" ("String") "deteccion" ("String") "espera" ("String") "movimiento" ("String")] -> w99
      tunnel: w98 -> [w411 _ _ _ _ _]
      tunnel: w97 -> [_ _ _ _ _ w675]
      tunnel: w96 -> [_ _ _ _ _ w674]
      tunnel: w95 -> [w406 w419 w469 w522 w582 w645]
      tunnel: w94 -> [_ _ _ _ _ w669]
      tunnel: w93 -> [_ _ _ _ _ w668]
      tunnel: w92 -> [w407 w420 w470 w521 w583 w666]
      tunnel: w91 -> [w410 w424 w474 w526 w585 w665]
      tunnel: w90 -> [w409 w423 w473 w525 w587 w664]
      tunnel: w89 -> [w408 w422 w472 w524 w586 w663]
      tunnel: [w405 w421 w471 w523 w584 w649] -> w88
      tunnel: [w410 w424 w474 w526 w585 w654] -> w87
      tunnel: [w407 w420 w470 w521 w583 w648] -> w86
      tunnel: [w409 w423 w473 w525 w587 w652] -> w85
      tunnel: [w408 w422 w472 w524 w586 w650] -> w84
      tunnel: [w406 w419 w469 w522 w582 w647] -> w83
      tunnel: w82 -> [_ _ _ _ _ w659]
      tunnel: w81 -> [_ _ _ _ _ w658]
      tunnel: w80 -> [w405 w421 w471 w523 w584 w656]
      tunnel: [FALSE w417 w468 w520 w581 w643] -> w57
      tunnel: [0.0 ("Duty Cycle") 0.94 ("Duty Cycle") 0.0 ("Duty Cycle") 0.94 ("Duty Cycle") 0.94 ("Duty Cycle") 0.0 ("Duty Cycle")] -> w27
      tunnel: [0.0 ("Duty Cycle") 0.94 ("Duty Cycle") 0.0 ("Duty Cycle") 0.0 ("Duty Cycle") 0.94 ("Duty Cycle") 0.0 ("Duty Cycle")] -> w26
      tunnel: w42 -> [_ _ _ w514 _ _]
      tunnel: w35 -> [_ _ _ _ _ _]
      tunnel: w33 -> [_ _ _ _ w574 _]
      frame "" {
      }
      frame "INICIO" {
        w417 = FALSE ("B/DIO2 (Pin 15)")
        n67 = case shown="True" "?" {
          tunnel: [T2."INICIO" T2."DETECCION"] -> w428
          frame False {
          }
          frame True {
          }
        }
        n68 = xnode "Digital output (1 sample) 8"("B/DIO2 (Pin 15)"=w417) -> ()  [unwired: 1 in, 1 out]
      }
      frame "STOP" {
        w468 = FALSE ("B/DIO2 (Pin 15)")
        n69 = xnode "Digital output (1 sample) 7"("B/DIO2 (Pin 15)"=w468) -> ()  [unwired: 1 in, 1 out]
      }
      frame "DETECCION" {
        w520 = FALSE ("B/DIO2 (Pin 15)")
        n70 = Or(x=w514, y="Boolean") -> (x .or. y?=w518:bool)
        n71 = case shown="True" w518 {
          tunnel: [T2."DETECCION" T2."ESPERA"] -> w532
          tunnel: [w569 w572] -> w531
          tunnel: w530 -> [w569 w572]
          tunnel: [w568 w571] -> w529
          tunnel: w528 -> [w568 w571]
          frame False {
          }
          frame True {
            # "1-6"
          }
        }
        n72 = xnode "Digital output (1 sample) 9"("B/DIO2 (Pin 15)"=w520) -> ()  [unwired: 1 in, 1 out]
        n73 = Wait (ms)(milliseconds to wait=u32 0) -> ()  [unwired: 1 out]
      }
      frame "ESPERA" {
        w581 = FALSE ("B/DIO2 (Pin 15)")
        n74 = Add(x=w592, y=1.0) -> (x+y=w576:dbl)
        n75 = Greater Or Equal?(x=w576, y=w574) -> (x >= y?=w577:bool)
        n76 = Select(t=0.0, s=w577, f=w576) -> (s? t:f=w588:dbl)
        n77 = case shown="False" w577 {
          tunnel: [T2."ESPERA" T2."MOVIMIENTO"] -> w591
          frame False {
          }
          frame True {
          }
        }
        n78 = xnode "Digital output (1 sample) 6"("B/DIO2 (Pin 15)"=w581) -> ()  [unwired: 1 in, 1 out]
        n79 = Wait (ms)(milliseconds to wait=u32 10) -> ()  [unwired: 1 out]
      }
      frame "MOVIMIENTO" {
        (unwired) 60.0 ("y")
        # "Ajustar"
        n80 = Add(x=w646, y="delta") -> (x+y=w680:dbl)
        n81 = call "lectura.vi"("Numeric in"=w663, "Numeric 3"=w664, "entrada1"=w665) -> ("Numeric 4"=w653:i32, "Real Matrix Element 2"=w636:dbl, "salida1"=w655:i32, "Numeric out"=w651:i32, "Real Matrix Element 3"=w637:dbl, "Real Matrix Element"=w635:dbl)  [unwired: 3 in]
        "POSICION1" <- w637
        "POSICION2" <- w636
        "POSICION3" <- w635
        "Slide" <- w637
        "Numeric" <- w637
        n82 = Greater Or Equal?(x=w637, y=36.0) -> (x >= y?=w641:bool)
        n83 = Less Or Equal?(x=w637, y=-130.0) -> ()  [unwired: 1 out]
        n84 = Greater Or Equal?(x=w680, y=7000.0) -> (x >= y?=w682:bool)
        n85 = Not(x=w641) -> (.not. x?=w643:bool)
        n86 = Wait (ms)(milliseconds to wait="velocidad") -> ()  [unwired: 1 out]
        n87 = call "subvimotor.vi"("PWM Ref Out"=w669, "error in (no error)"=w668, "freq [Hz] 3"=50.0, "null offset 3"="null offset 4", "position [%FS] 3"=w666) -> ("Numeric"=→"duty cycle [%] 4":dbl, "Numeric 2"=→"pulse width [ms] 4":dbl, "position [%FS]"=→"offset [%FS] 4" →"position [%FS]":dbl)  [unwired: 4 in]
        n88 = shared-variable "miRIO1\\VARIABLE_COMPARTIDA.lvlib\\ZPOS"(w635) -> ()  [unwired: 1 in, 1 out]
        n89 = Select(t=0.0, s=w682, f=w680) -> (s? t:f=w679:dbl)
        n90 = call "subvimotor.vi"("PWM Ref Out"=w675, "error in (no error)"=w674, "freq [Hz] 3"=50.0, "null offset 3"="null offset 3", "position [%FS] 3"=w645) -> ("Numeric"=→"duty cycle [%] 3":dbl, "Numeric 2"=→"pulse width [ms] 3":dbl, "position [%FS]"=→"offset [%FS] 3" →"position [3":dbl)  [unwired: 4 in]
        n91 = call "subvimotor.vi"("PWM Ref Out"=w659, "error in (no error)"=w658, "freq [Hz] 3"=50.0, "null offset 3"="null offset 5", "position [%FS] 3"=w656) -> ("Numeric"=→"duty cycle [%] 5":dbl, "Numeric 2"=→"pulse width [ms] 5":dbl, "position [%FS]"=→"offset [%FS] 5" →"position1":dbl)  [unwired: 4 in]
        n92 = case shown="False" w682 {
          tunnel: [T2."MOVIMIENTO" T2."INICIO"] -> w686
          tunnel: [w764 w772] -> w685
          tunnel: w684 -> [w764 w772]
          tunnel: w655 -> [w763 _]
          tunnel: [w763 -1] -> w654
          tunnel: w653 -> [w762 _]
          tunnel: [w762 -1] -> w652
          tunnel: w651 -> [w761 _]
          tunnel: [w761 -1] -> w650
          tunnel: w637 -> [w760 _]
          tunnel: [w760 0.0 ("t")] -> w649
          tunnel: w636 -> [w759 _]
          tunnel: [w759 0.0 ("t")] -> w648
          tunnel: w635 -> [w758 _]
          tunnel: [w758 0.0 ("t")] -> w647
          frame False {
          }
          frame True {
          }
        }
        n93 = xnode "Digital output (1 sample) 5"("B/DIO2 (Pin 15)"=w643) -> ()  [unwired: 1 in, 1 out]
        n94 = shared-variable "miRIO1\\VARIABLE_COMPARTIDA.lvlib\\YPOS"(w636) -> ()  [unwired: 1 in, 1 out]
        n95 = shared-variable "miRIO1\\VARIABLE_COMPARTIDA.lvlib\\XPOS"(w637) -> ()  [unwired: 1 in, 1 out]
        n96 = xnode "Digital output (1 sample)"("A/DIO1 (Pin 13)"=w643) -> ()  [unwired: 1 in, 1 out]
      }
    }
    "ESTADO" <- w99
    "ventosa" <- w57
    n97 = Match Pattern(string=w74, regular expression="CH0") -> (after substring=w76:string)  [unwired: 1 in, 3 out]
    n98 = Match Pattern(string=w74, regular expression="CH1") -> (after substring=w75:string)  [unwired: 1 in, 3 out]
    n99 = Fract/Exp String To Number(string=w76) -> (number=w72:dbl)  [unwired: 3 in, 1 out]
    "CADENA1" <- w72
    n100 = Fract/Exp String To Number(string=w75) -> (number=w67:dbl)  [unwired: 3 in, 1 out]
    "CADENA2" <- w67
    n101 = Select(t=1.0, s=w42, f=0.0) -> (s? t:f=w48:dbl)
    n102 = Greater Or Equal?(x=w67, y=10.0) -> ()  [unwired: 1 out]
    n103 = Bundle(w72, w67) -> (→"Datos recibidos vía TCP":cluster{dbl, dbl})  [unwired: 1 in]
    n104 = Subtract(x=w35, y=w48) -> (x-y=w49:dbl)
    n105 = Equal?(x=w49, y=1.0) -> (x = y?=w54:bool)
    n106 = case shown="True" w54 {
      tunnel: [w107 29.0] -> w50
      tunnel: w49 -> [w107 _]
      frame False {
      }
      frame True {
      }
    }
    n107 = shared-variable "miRIO1\\VARIABLE_COMPARTIDA.lvlib\\PARADADATO"() -> (w55:bool)  [unwired: 1 in, 1 out]
    n108 = Multiply(x=w27, y=100.0) -> (x*y=w24:dbl)
    n109 = shared-variable "miRIO1\\VARIABLE_COMPARTIDA.lvlib\\MOTOR2"(w24) -> ()  [unwired: 1 in, 1 out]
    n110 = xnode "PWM 7"("Duty Cycle"=w26) -> ()  [unwired: 1 in, 1 out]
    n111 = xnode "PWM 8"("Duty Cycle"=w27) -> ()  [unwired: 1 in, 1 out]
    n112 = Multiply(x=w26, y=100.0) -> (x*y=w25:dbl)
    n113 = Compound Arithmetic op=OR(w55, "PARADA", "PARADA", "PARADA", "PARADA") -> (w56:bool)
    n114 = shared-variable "miRIO1\\VARIABLE_COMPARTIDA.lvlib\\MOTOR1"(w25) -> ()  [unwired: 1 in, 1 out]
    n115 = shared-variable "miRIO1\\VARIABLE_COMPARTIDA.lvlib\\PARADA"(w55) -> ()  [unwired: 1 in, 1 out]
    "Numeric 5" <- w35
  }
  n116 = call <vilib>:"Simple Error Handler.vi"() -> ("error out"=w23:errorcluster)  [unwired: 5 in, 4 out]
  n117 = call <vilib>:"Reset myRIO.vi"("error in (no error)"=w23) -> ()  [unwired: 10 in, 1 out]
